vi "Tools_String Remap EOLN.vi"(0 "string in":string, 1 "line separator (\\r\\n)":string="\r\n") -> (2 "string out":string)   [LabVIEW 2017]
doc: "Replaces all EOLN characters in the string with \"line separator\"."
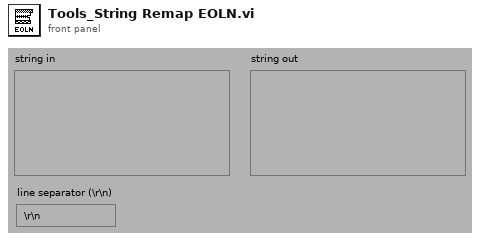
[diagram p1: front panel]
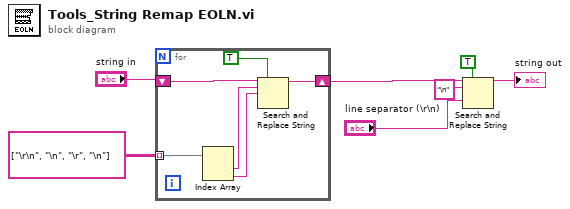
[diagram p0: block diagram]
diagram:
  n1 = for {
    tunnel: string[][] [["\r\n", "\n"], ["\r", "\n"]] -> [w13] mode=indexing
    shift-right: [w9] -> w2
    shift-left: "string in" -> [w12]
    n2 = Index Array(array=w13) -> (element #1=w11:string, element #2=w10:string)  [unwired: 2 in]
    n3 = Search and Replace String(replace all?=TRUE ("replace all? (F)"), input string=w12, search string=w11, replace string=w10) -> (result string=w9:string)  [unwired: 1 in, 6 out]
  }
  n4 = Search and Replace String(replace all?=TRUE ("replace all? (F)"), input string=w2, search string="\n", replace string="line separator (\\r\\n)") -> (result string=→"string out":string)  [unwired: 1 in, 6 out]
